vi "CMD_Drive.vi"(1 "Line":string) -> (0 "Done":bool=TRUE)   [LabVIEW 2017, in "Apple script.lvlib"]
uses:
  Apple script.lvlib
  Robot Global Data.vi
  <vilib>/addons/control/pid/pid.llb/PID (DBL).vi
  <vilib>/Rock Robotics/Network Tables/NT Write Numeric Array.vi
  <vilib>/addons/control/pid/NI_PID_pid.lvlib
  Support Code/Support Code.lvlib
panel:
  in  "Angle PID":T1={"proportional gain (Kc)"=0.025, "integral time (Ti, min)"=0.0, "derivative time (Td, min)"=0.0}
  in  "Y gains":T1={"proportional gain (Kc)"=0.325, "integral time (Ti, min)"=0.0, "derivative time (Td, min)"=0.0}
  in  "x 2":dbl=0.1 format="%#_13g"
  in  "X PID":T1={"proportional gain (Kc)"=0.325, "integral time (Ti, min)"=0.0, "derivative time (Td, min)"=0.0}
  in  "Subcommands":string[](array[string])=["at", "at", "for", "to", "until", "to"]
  in  "Parameters":i32[](array[numeric])=[1, 3, 1, 3, 1, 2]
  # "try changing execution\ntype"
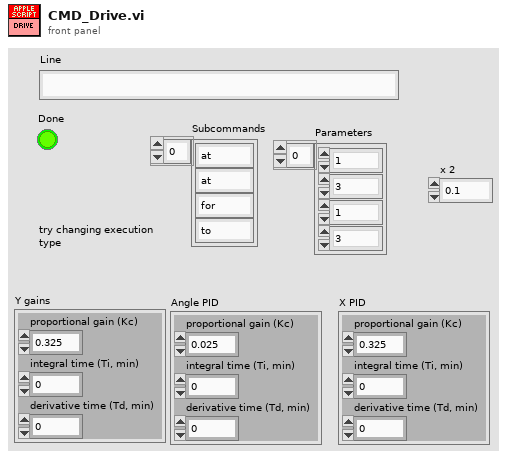
[diagram p1: front panel]
types:
  T1 = cluster{"proportional gain (Kc)":dbl, "integral time (Ti, min)":dbl, "derivative time (Td, min)":dbl}
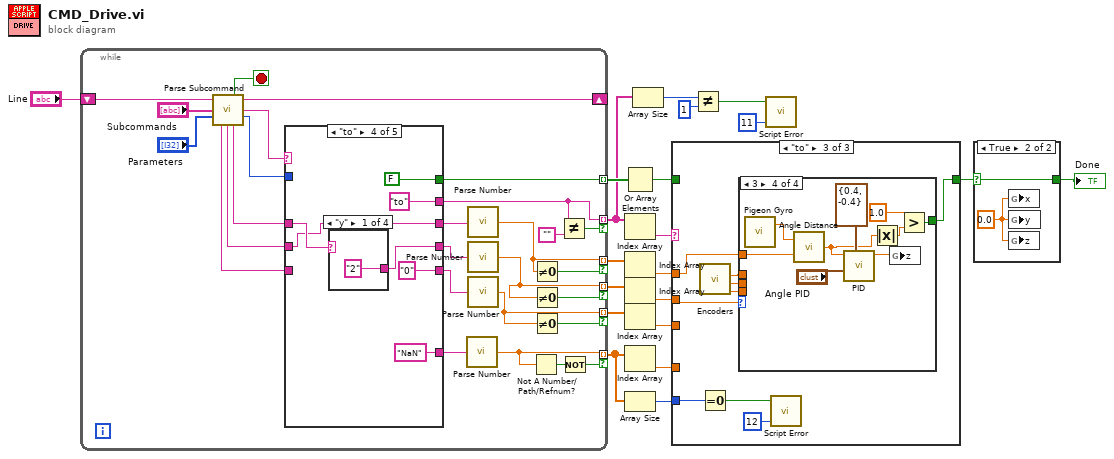
[diagram p0: block diagram]
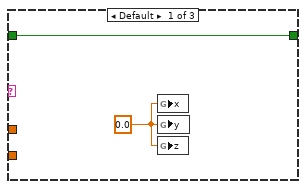
[diagram p3: hidden frame]
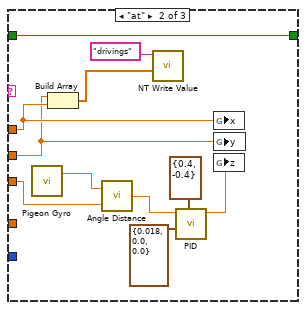
[diagram p4: hidden frame]
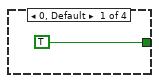
[diagram p5: hidden frame]
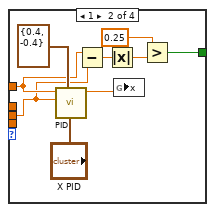
[diagram p6: hidden frame]
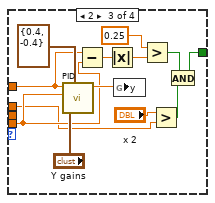
[diagram p7: hidden frame]
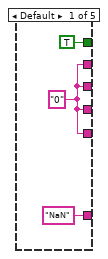
[diagram p8: hidden frame]
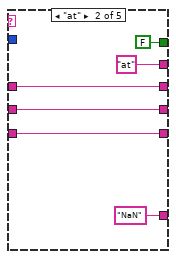
[diagram p9: hidden frame]
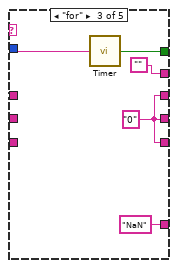
[diagram p10: hidden frame]
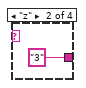
[diagram p11: hidden frame]
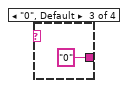
[diagram p12: hidden frame]
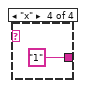
[diagram p13: hidden frame]
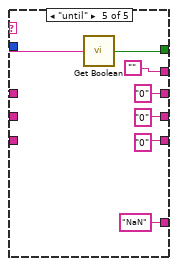
[diagram p14: hidden frame]
diagram:
  n1 = while {
    shift-right: [w44] -> _
    shift-left: "Line" -> [w47]
    tunnel: [w22] -> w6 mode=indexing
    tunnel: [w34] -> w18 mode=indexing if=w28
    tunnel: [w33] -> w16 mode=indexing if=w26
    tunnel: [w30] -> w14 mode=indexing if=w27
    tunnel: [w25] -> w4 mode=indexing if=w23
    tunnel: [w21] -> w5 mode=indexing if=w36
    stop <- w43 stop-if-true
    n2 = call "Parse Subcommand.vi"("Text In"=w47, "Subcommands"="Subcommands", "Parameters"="Parameters") -> ("Done"=w43:bool, "Text Out"=w44:string, "Subcommand"=w42:string, "# of Parameters"=w41:i32, "Parameter 3"=w39:string, "Parameter 2"=w38:string, "Parameter 1"=w40:string)  [unwired: 6 in]
    n3 = case shown="\"to\"" w42 {
      tunnel: w41 -> [_ _ _ _ _]
      tunnel: w40 -> [_ w56 w58 w66 w74]
      tunnel: w38 -> [_ w55 _ w65 _]
      tunnel: w39 -> [_ w54 _ _ _]
      tunnel: [w49 w56 w57 w65 "0" ("Parameter 1")] -> w35
      tunnel: [w49 w55 w57 w64 "0" ("Parameter 1")] -> w32
      tunnel: [w49 w54 w57 "0" ("Parameter 3") "0" ("Parameter 1")] -> w31
      tunnel: [TRUE ("Value") FALSE ("Running") w59 FALSE w73] -> w22
      tunnel: [w49 "at" "" "to" ("format string") ""] -> w21
      tunnel: ["NaN" ("Parameter 1") "NaN" ("Parameter 3") "NaN" ("Parameter 3") "NaN" ("Parameter 3") "NaN" ("Parameter 1")] -> w29
      frame Default {
        w49 = "0" ("format string")
      }
      frame "at" {
      }
      frame "for" {
        w57 = "0" ("Parameter 1")
        n4 = call "Timer.vi"("Seconds (string)"=w58) -> ("Done"=w59:bool)
      }
      frame "to" {
        n5 = case shown="\"y\"" w66 {
          tunnel: ["2" "3" "0" "1"] -> w64
          frame "y" {
          }
          frame "z" {
          }
          frame "0", Default {
          }
          frame "x" {
          }
        }
      }
      frame "until" {
        n6 = call "Get Boolean.vi"("Name"=w74) -> ("Value"=w73:bool)
      }
    }
    n7 = call "Parse Number.vi"("String"=w29) -> ("Number"=w25:dbl)
    n8 = call "Parse Number.vi"("String"=w35) -> ("Number"=w34:dbl)
    n9 = call "Parse Number.vi"("String"=w32) -> ("Number"=w33:dbl)
    n10 = call "Parse Number.vi"("String"=w31) -> ("Number"=w30:dbl)
    n11 = Not A Number/Path/Refnum?(number/path/refnum=w25) -> (NaN/Path/Refnum?=w24:bool)
    n12 = Not Equal To 0?(x=w34) -> (x != 0?=w28:bool)
    n13 = Not Equal To 0?(x=w33) -> (x != 0?=w26:bool)
    n14 = Not Equal To 0?(x=w30) -> (x != 0?=w27:bool)
    n15 = Not Equal?(x=w21, y="") -> (x != y?=w36:bool)
    n16 = Not(x=w24) -> (.not. x?=w23:bool)
  }
  n17 = Or Array Elements(Boolean array=w6) -> (logical OR=w2:bool)
  n18 = Index Array(array=w5) -> (element=w11:string)  [unwired: 1 in]
  n19 = Index Array(array=w18) -> (element=w17:dbl)  [unwired: 1 in]
  n20 = Index Array(array=w16) -> (element=w15:dbl)  [unwired: 1 in]
  n21 = Index Array(array=w14) -> (element=w13:dbl)  [unwired: 1 in]
  n22 = Index Array(array=w4) -> (element=w12:dbl)  [unwired: 1 in]
  n23 = Array Size(array=w4) -> (size(s)=w3:i32)
  n24 = Array Size(array=w5) -> (size(s)=w9:i32)
  n25 = case shown="\"to\"" w11 {
    tunnel: w17 -> [_ w85 w94]
    tunnel: w2 -> [w81 w92 _]
    tunnel: [w81 w92 w93] -> w1
    tunnel: w15 -> [_ w84 w95]
    tunnel: w13 -> [_ w88 _]
    tunnel: w12 -> [_ _ _]
    tunnel: w3 -> [_ _ w100]
    frame Default {
      w80 = 0.0 ("X")
      n26 = global write "Robot Global Data.vi" "x"(w80) -> ()
      n27 = global write "Robot Global Data.vi" "y"(w80) -> ()
      n28 = global write "Robot Global Data.vi" "z"(w80) -> ()
    }
    frame "at" {
      n29 = call "Pigeon Gyro.vi"() -> ("YPR.Yaw"=w89:dbl)  [unwired: 1 in, 1 out]
      n30 = Build Array(w84, w85) -> (w82:dbl[])
      n31 = call "Angle Distance.vi"("target angle"=w88, "current angle"=w89) -> ("distance"=w87:dbl)
      n32 = call-poly <vilib>:"NT Write Value.vi"("Numeric Array"=w82, "Name"="drivings") -> ()  [unwired: 9 in, 1 out]
      n33 = call-poly <vilib>:"PID.vi"("output range"=cluster{"output high":dbl, "output low":dbl} {"output high"=0.4, "output low"=-0.4}, "PID gains"=T1 {"proportional gain (Kc)"=0.018, "integral time (Ti, min)"=0.0, "derivative time (Td, min)"=0.0}, "setpoint"=w87) -> ("output"=w83:dbl)  [unwired: 7 in, 1 out]
      n34 = global write "Robot Global Data.vi" "x"(w85) -> ()
      n35 = global write "Robot Global Data.vi" "y"(w84) -> ()
      n36 = global write "Robot Global Data.vi" "z"(w83) -> ()
    }
    frame "to" {
      n37 = call "Encoders.vi"() -> ("Avg Rate"=w96:dbl, "X Distance"=w98:dbl, "Y Distance"=w97:dbl)  [unwired: 3 in, 1 out]
      n38 = Equal To 0?(x=w100) -> (x = 0?=w99:bool)
      n39 = case shown="3" w95 {
        tunnel: [TRUE ("Done") w103 w114 w125] -> w93
        tunnel: w98 -> [_ w107 _ _]
        tunnel: w97 -> [_ _ w121 _]
        tunnel: w94 -> [_ w108 w120 w129]
        tunnel: w96 -> [_ _ w112 _]
        frame 0, Default {
        }
        frame 1 {
          n40 = call-poly <vilib>:"PID.vi"("output range"=cluster{"output high":dbl, "output low":dbl} {"output high"=0.4, "output low"=-0.4}, "PID gains"="X PID", "process variable"=w107, "setpoint"=w108) -> ("output"=w111:dbl)  [unwired: 6 in, 1 out]
          n41 = Subtract(x=w108, y=w107) -> (x-y=w106:dbl)
          n42 = Absolute Value(x=w106) -> (abs(x)=w105:dbl)
          n43 = global write "Robot Global Data.vi" "x"(w111) -> ()
          n44 = Greater?(x=0.25, y=w105) -> (0:w103:bool)
        }
        frame 2 {
          n45 = call-poly <vilib>:"PID.vi"("output range"=cluster{"output high":dbl, "output low":dbl} {"output high"=0.4, "output low"=-0.4}, "PID gains"="Y gains", "process variable"=w121, "setpoint"=w120) -> ("output"=w124:dbl)  [unwired: 6 in, 1 out]
          n46 = Subtract(x=w120, y=w121) -> (x-y=w117:dbl)
          n47 = Absolute Value(x=w117) -> (abs(x)=w118:dbl)
          n48 = global write "Robot Global Data.vi" "y"(w124) -> ()
          n49 = Greater?(x=0.25, y=w118) -> (0:w115:bool)
          n50 = Greater?(x="x 2", y=w112) -> (0:w116:bool)
          n51 = And(x=w115, y=w116) -> (x .and. y?=w114:bool)
        }
        frame 3 {
          n52 = call "Pigeon Gyro.vi"() -> ("YPR.Yaw"=w130:dbl)  [unwired: 1 in, 1 out]
          n53 = call "Angle Distance.vi"("target angle"=w129, "current angle"=w130) -> ("distance"=w128:dbl)
          n54 = call-poly <vilib>:"PID.vi"("output range"=cluster{"output high":dbl, "output low":dbl} {"output high"=0.4, "output low"=-0.4}, "PID gains"="Angle PID", "setpoint"=w128) -> ("output"=w133:dbl)  [unwired: 7 in, 1 out]
          n55 = Absolute Value(x=w128) -> (abs(x)=w126:dbl)
          n56 = global write "Robot Global Data.vi" "z"(w133) -> ()
          n57 = Greater?(x=1.0, y=w126) -> (0:w125:bool)
        }
      }
      n58 = call "Script Error.vi"("Error?"=w99, "Error Code"=12) -> ()  [unwired: 3 in, 1 out]
    }
  }
  n59 = Not Equal?(x=w9, y=1) -> (x != y?=w7:bool)
  n60 = call "Script Error.vi"("Error?"=w7, "Error Code"=11) -> ()  [unwired: 3 in, 1 out]
  n61 = case shown="True" w1 {
    selector: w1 -> [w134 w136]
    tunnel: [w134 w136] -> w19
    frame False {
    }
    frame True {
      w135 = 0.0 ("X")
      n62 = global write "Robot Global Data.vi" "x"(w135) -> ()
      n63 = global write "Robot Global Data.vi" "y"(w135) -> ()
      n64 = global write "Robot Global Data.vi" "z"(w135) -> ()
    }
  }
  "Done" <- w19
